vi "GetTreeIndentLevel0.vi"(11 "Tree 2":refnum<vi>) -> (3 "Indent Level 0":string[](array[string]))   [LabVIEW 2025]
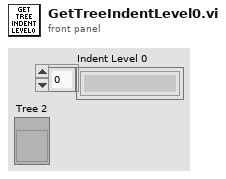
[diagram p1: front panel]
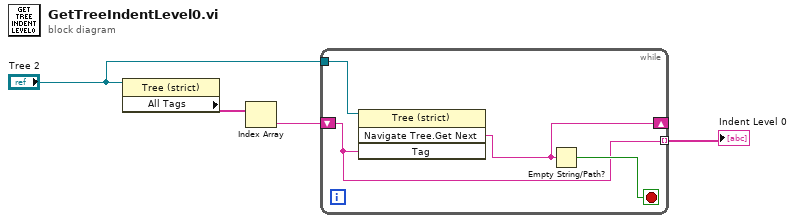
[diagram p0: block diagram]
diagram:
  n1 = property class="Tree (strict)"(reference="Tree 2") -> ("All Tags"=w4:string[])  [unwired: 1 in, 2 out]
  n2 = Index Array(array=w4) -> (element=w3:string)  [unwired: 1 in]
  n3 = while {
    shift-right: [w7] -> _
    shift-left: w3 -> [w5]
    tunnel: "Tree 2" -> [w8]
    tunnel: [w5] -> w2 mode=indexing
    stop <- w6 stop-if-true
    n4 = invoke class="Tree (strict)" method="Navigate Tree.Get Next"(reference=w8, "Tag"=w5) -> ("Navigate Tree:Get Next Item"=w7:string)  [unwired: 2 in, 3 out]
    n5 = Empty String/Path?(string/path=w7) -> (empty?=w6:bool)
  }
  "Indent Level 0" <- w2
